vi "MtAtElectrometer_logEvent_measureRange.vi"(8 "error in (no error)":errorcluster, 11 "logevent_measureRange_Ctl":T1) -> (0 "error out":errorcluster, 2 "function return":i32, 3 "logevent_measureRange_Ctl out":T1)   [LabVIEW 2016, in "SALLV_MtAtElectrometer.lvlib"]
doc: "int MtAtElectrometer_shm_logEvent_measureRangeLV(MtAtElectrometer_logevent_measureRangeLV *logevent_measureRange_Ctl );"
uses:
  SALLV_MtAtElectrometer.lvlib
  DataTypes/logevent_measureRange.ctl
  ts_sal/test/MtAtElectrometer/labview/SALLV_MtAtElectrometer.so
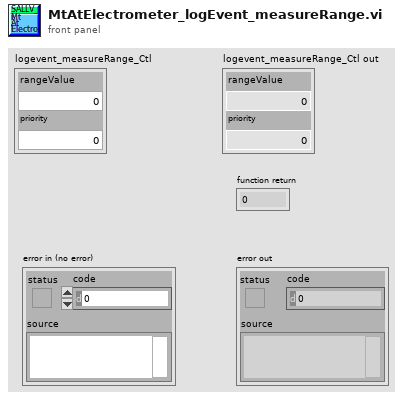
[diagram p1: front panel]
types:
  T1 = typedef "SALLV_MtAtElectrometer.lvlib/logevent_measureRange.ctl" = cluster{"rangeValue":dbl, "priority":i32}
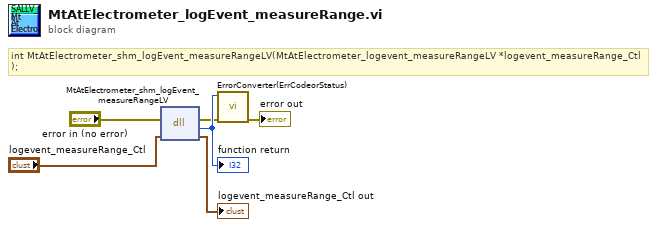
[diagram p0: block diagram]
diagram:
  # "int MtAtElectrometer_shm_logEvent_measureRangeLV(MtAtElectrometer_logevent_measureRangeLV *logevent_measureRange_Ctl );"
  n1 = dll-call lib="home/andres/ts_sal/test/MtAtElectrometer/labview/SALLV_MtAtElectrometer.*" fn="MtAtElectrometer_shm_logEvent_measureRangeLV"(error in="error in (no error)", "logevent_measureRange_Ctl"="logevent_measureRange_Ctl") -> (error out=w2:errorcluster, w6:i32, "logevent_measureRange_Ctl"=→"logevent_measureRange_Ctl out":T1)  [unwired: 2 in, 1 out]
  "function return" <- w6
  n2 = call "ErrorConverter(ErrCodeorStatus).vi"("error in (no error)"=w2, "error code"=w6) -> ("error out"=→"error out":errorcluster)  [unwired: 9 in]
